vi "Moxom Run (RT RHIT's conflicted copy 2012-03-21).vi"() -> ()   [LabVIEW 2011]
uses:
  <vilib>/Instr/_visa.llb/VISA Configure Serial Port (Instr).vi
  <vilib>/Utility/inputDevices.llb/joystickAcquire.vi
panel:
  out "Numeric 2":i32
  out "Numeric":i32
  in  "Durration":i32[](array[numeric])
  in  "Right Motor":i32[](array[numeric])
  in  "Left Motor":i32[](array[numeric])
  in  "Motor Controller\nSerial Port":refnum<visa-resource-name>
  out "Right Motor Remote":i32
  out "Right Motor Auto":i32
  out "Left Motor Remote":i32
  out "Left Motor Auto":i32
  out "Auto Enabled":bool
  in  "Auto":bool
  in  "stop":bool
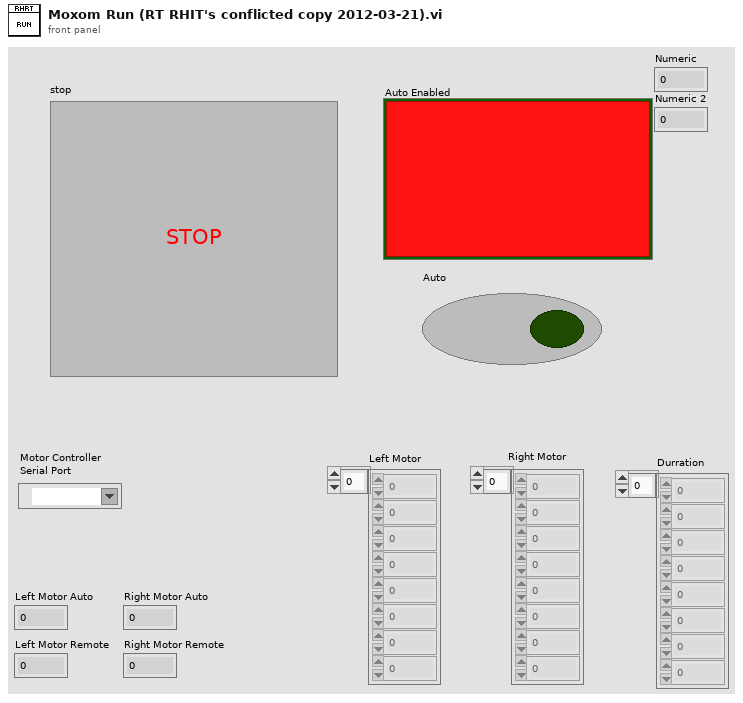
[diagram p1: front panel]
types:
  T1 = cluster{"axes total":u32, "buttons total":u32, "pov total":u32, "device name":string}[]
  T2 = cluster{"button 1":bool, "button 2":bool, "button 3":bool, "button 4":bool, "button 5":bool, "button 6":bool, "button 7":bool, "button 8":bool, "button 9":bool, "button 10":bool, "button 11":bool, "button 12":bool, "button 13":bool, "button 14":bool, "button 15":bool, "button 16":bool, "button 17":bool, "button 18":bool, "button 19":bool, "button 20":bool, "button 21":bool, "button 22":bool, "button 23":bool, "button 24":bool, "button 25":bool, "button 26":bool, "button 27":bool, "button 28":bool, "button 29":bool, "button 30":bool, "button 31":bool, "button 32":bool}
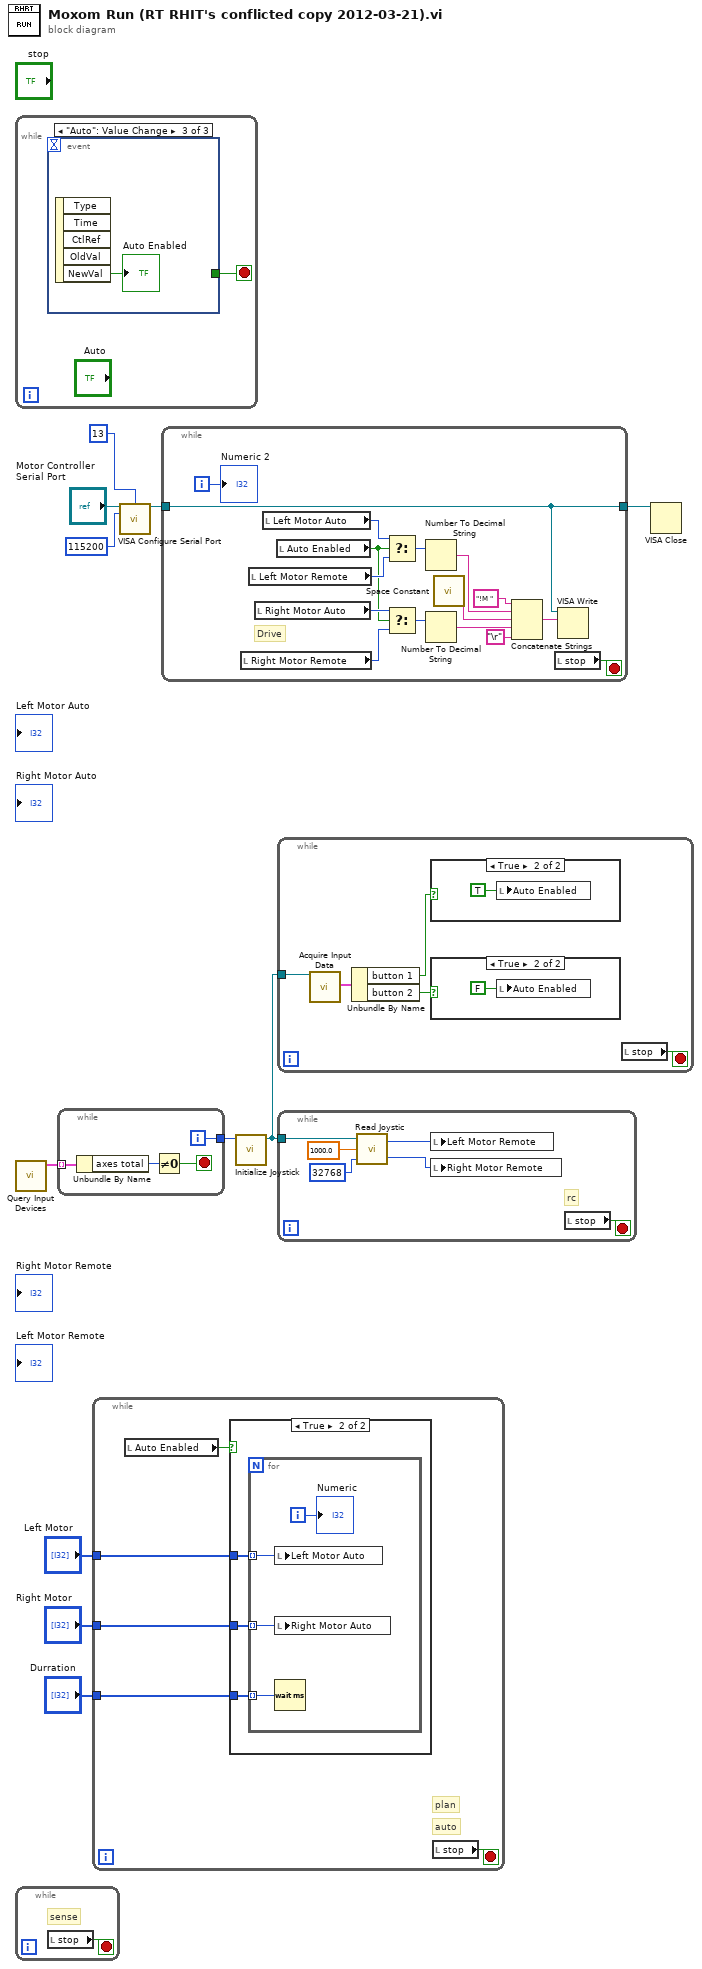
[diagram p0: block diagram]
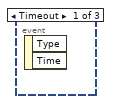
[diagram p5: hidden frame]
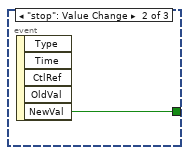
[diagram p6: hidden frame]
diagram:
  n1 = while {
    stop <- w12 stop-if-true
    n2 = event shown="[2] \"Auto\": Value Change" {
      selector: _ -> [_ _ _]
      dyn-events: _ -> [_ _ _]
      timeout: _ -> [_ _ _]
      tunnel: [_ w13 _] -> w12
      event Timeout {
        n3 = event-data() -> ()  [unwired: 1 in, 2 out]
      }
      event "stop": Value Change {
        n4 = event-data() -> ("NewVal"=w13:bool)  [unwired: 1 in, 4 out]
      }
      event "Auto": Value Change {
        n5 = event-data() -> ("NewVal"=→"Auto Enabled":bool)  [unwired: 1 in, 4 out]
      }
    }
  }
  n6 = call <vilib>:"Query Input Devices.vi"() -> ("joystick info"=w3:T1)  [unwired: 8 in, 3 out]
  n7 = while {
    stop <- w15 stop-if-true
    # "sense"
    n8 = local read "stop"() -> (w15:bool)
  }
  n9 = while {
    tunnel: w3 -> [w19] mode=indexing
    tunnel: [w16] -> w2
    i -> [w16]
    stop <- w17 stop-if-true
    n10 = Unbundle By Name(w19) -> ("axes total"=w18:u32)
    n11 = Not Equal To 0?(x=w18) -> (x != 0?=w17:bool)
  }
  n12 = while {
    tunnel: "Left Motor" -> [w22]
    tunnel: "Right Motor" -> [w21]
    tunnel: "Durration" -> [w20]
    stop <- w24 stop-if-true
    # "auto"
    # "plan"
    n13 = local read "Auto Enabled"() -> (w23:bool)
    n14 = case shown="True" w23 {
      tunnel: w22 -> [_ w27]
      tunnel: w21 -> [_ w26]
      tunnel: w20 -> [_ w25]
      frame False {
      }
      frame True {
        n15 = for {
          tunnel: w27 -> [w30] mode=indexing
          tunnel: w26 -> [w29] mode=indexing
          tunnel: w25 -> [w31] mode=indexing
          i -> [w28]
          n16 = local write "Left Motor Auto"(w30) -> ()
          n17 = local write "Right Motor Auto"(w29) -> ()
          n18 = Wait (ms)(milliseconds to wait=w31) -> ()  [unwired: 1 out]
          "Numeric" <- w28
        }
      }
    }
    n19 = local read "stop"() -> (w24:bool)
  }
  n20 = call-poly "VISA Configure Serial Port"("VISA resource name"="Motor Controller\nSerial Port", "termination char\n(0xA = '\\n' = LF)"=u8 13 ("termination char\n(0xA = '\\n' = LF)"), "baud rate (9600)"=u32 115200) -> ("VISA resource name out"=w8:refnum<visa-resource-name>)  [unwired: 11 in, 1 out]
  n21 = while {
    tunnel: w8 -> [w32]
    tunnel: [w32] -> w7
    i -> [w37]
    stop <- w47 stop-if-true
    # "Drive"
    n22 = local read "Right Motor Remote"() -> (w43:i32)
    n23 = local read "Left Motor Remote"() -> (w45:i32)
    n24 = local read "Right Motor Auto"() -> (w44:i32)
    n25 = local read "Left Motor Auto"() -> (w46:i32)
    n26 = local read "Auto Enabled"() -> (w42:bool)
    n27 = Select(t=w46, s=w42, f=w45) -> (s? t:f=w38:i32)
    n28 = Select(t=w44, s=w42, f=w43) -> (s? t:f=w39:i32)
    n29 = Number To Decimal String(number=w38) -> (decimal integer string=w36:string)  [unwired: 1 in]
    n30 = Number To Decimal String(number=w39) -> (decimal integer string=w35:string)  [unwired: 1 in]
    n31 = call <vilib>:"Space Constant.vi"() -> ("String"=w40:string)
    n32 = Concatenate Strings("!M " ("string"), w36, w40, w35, "\r") -> (w33:string)
    n33 = local read "stop"() -> (w47:bool)
    n34 = VISA Write(VISA resource name=w32, write buffer=w33) -> ()  [unwired: 1 in, 3 out]
    "Numeric 2" <- w37
  }
  n35 = call <vilib>:"Initialize Joystick.vi"("device index"=w2) -> ("device ID"=w1:refnum<k1>)  [unwired: 9 in, 1 out]
  n36 = while {
    tunnel: w1 -> [w52]
    stop <- w48 stop-if-true
    n37 = call-poly <vilib>:"Acquire Input Data.vi"("device ID"=w52) -> ("button info"=w51:T2)  [unwired: 14 in, 4 out]
    n38 = Unbundle By Name(w51) -> ("button 1"=w50:bool, "button 2"=w49:bool)
    n39 = case shown="True" w50 {
      frame False {
      }
      frame True {
        n40 = local write "Auto Enabled"(TRUE ("Auto Enabled")) -> ()
      }
    }
    n41 = case shown="True" w49 {
      frame False {
      }
      frame True {
        n42 = local write "Auto Enabled"(FALSE ("Auto Enabled")) -> ()
      }
    }
    n43 = local read "stop"() -> (w48:bool)
  }
  n44 = while {
    tunnel: w1 -> [w55]
    stop <- w60 stop-if-true
    # "rc"
    n45 = call "Read Joystic.vi"("JoystickOutMaximum"=32768, "MaxMotorSpeed"=1000.0 ("HalfMaxMotorSpeed"), "device ID"=w55) -> ("Right Motor"=w56:i32, "Left Motor"=w57:i32)
    n46 = local write "Left Motor Remote"(w57) -> ()
    n47 = local write "Right Motor Remote"(w56) -> ()
    n48 = local read "stop"() -> (w60:bool)
  }
  n49 = VISA Close(VISA resource name=w7) -> ()  [unwired: 1 in, 1 out]
